vi "Serial.FrameSend.vi"(0 "VISA resource name":refnum<visa-resource-name> caption="Serial Port", 1 "timeout (10sec)":u32=1000 caption="超时（10秒）", 5 "baud rate (9600)":u32=9600 caption="波特率(9600)", 7 "写入缓冲区":string, 9 "写入字节数组":u8[](array[numeric]) format="%02x", 11 "error in (no error)":errorcluster caption="错误输入（无错误）", 12 "Send Mode":enum16{"0-发送文本", "1-发送16进制数组"}(ring)) -> (4 "Success?":bool, 10 "HEX字符串":string, 15 "error out":errorcluster caption="错误输出")   [LabVIEW 2012, in "Lib_UEL.ATE.lvlib" / "Lib_2Voice.lvlib"]
uses:
  Lib_2Voice.lvlib
  <vilib>/Instr/_visa.llb/VISA Configure Serial Port (Instr).vi
panel:
  # "V001 - Initial Version. ~LI.Guang 2015-11-10"
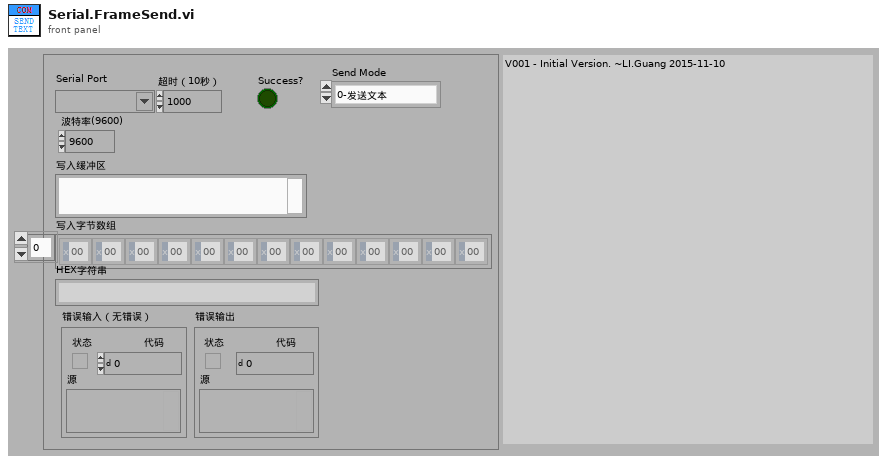
[diagram p1: front panel]
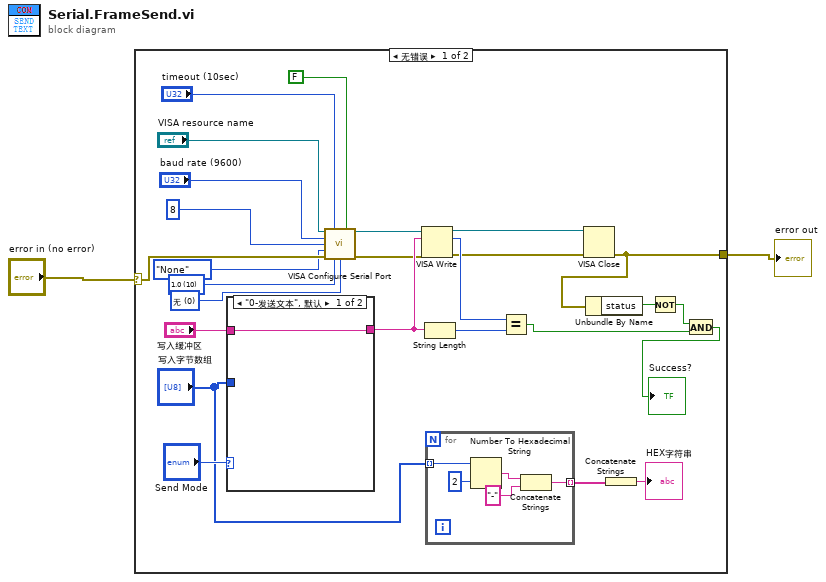
[diagram p0: block diagram]
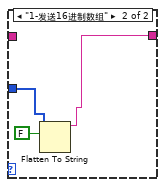
[diagram p2: hidden frame]
diagram:
  n1 = case shown="无错误" "error in (no error)" {
    selector: "error in (no error)" -> [w25 w38]
    tunnel: [w20 w38] -> w1
    frame No Error {
      w7 = u16 0 items=["无", "XON/XOFF", "RTS/CTS", "XON/XOFF & RTS/CTS", "DTR/DSR", "XON/XOFF & DTR/DSR"] ("flow control (0:none)")
      w8 = u16 10 items=["1.0"=10, "1.5"=15, "2.0"=20] ("stop bits (10: 1 bit)")
      n2 = case shown="\"0-发送文本\", 默认" "Send Mode" {
        tunnel: "写入字节数组" -> [_ w37]
        tunnel: [w34 w36] -> w16
        tunnel: "写入缓冲区" -> [w34 _]
        frame "0-发送文本", Default {
        }
        frame "1-发送16进制数组" {
          n3 = Flatten To String(anything=w37, prepend array or string size? (T)=FALSE ("预置数组或字符串大小？(T)")) -> (data string=w36:string)  [unwired: 2 in, 2 out]
        }
      }
      n4 = call-poly "VISA Configure Serial Port"("VISA resource name"="VISA resource name", "timeout (10sec)"="timeout (10sec)", "Enable Termination\nChar (T)"=FALSE ("Disable Termination\nChar (T)"), "baud rate (9600)"="baud rate (9600)", "data bits (8)"=u16 8, "parity (0:none)"=enum16{"None", "Odd", "Even", "Mark", "Space"}."None", "error in (no error)"=w25, "stop bits (10: 1 bit)"=w8, "flow control (0:none)"=w7) -> ("VISA resource name out"=w4:refnum<visa-resource-name>, "error out"=w3:errorcluster)  [unwired: 5 in]
      n5 = VISA Write(VISA resource name=w4, write buffer=w16, error in (no error)=w3) -> (VISA resource name out=w6:refnum<visa-resource-name>, return count=w23:u32, error out=w5:errorcluster)
      n6 = String Length(string=w16) -> (length=w24:i32)
      n7 = for {
        tunnel: "写入字节数组" -> [w33] mode=indexing
        tunnel: [w29] -> w13 mode=indexing
        n8 = Number To Hexadecimal String(1:i16 2 ("宽度(-)"), 2:w33) -> (0:w31:string)
        n9 = Concatenate Strings(w31, "-" ("字符串")) -> (w29:string)
      }
      n10 = Equal?(x=w23, y=w24) -> (x = y?=w19:bool)
      n11 = VISA Close(VISA resource name=w6, error in (no error)=w5) -> (error out=w20:errorcluster)
      n12 = Unbundle By Name(w20) -> ("status"=w21:bool)
      n13 = Concatenate Strings(w13) -> (→"HEX字符串":string)
      n14 = Not(x=w21) -> (.not. x?=w22:bool)
      n15 = And(x=w22, y=w19) -> (x .and. y?=→"Success?":bool)
    }
    frame Error {
    }
  }
  "error out" <- w1
